vi "{{Name}}.vi"(6 "Error":errorcluster, 7 "Message":refnum<class "Message.lvclass">, 11 "ConcreteMessage":refnum<class "ConcreteMessage.lvclass">) -> (3 "ConcreteMessage":refnum<class "ConcreteMessage.lvclass">, 4 "Error":errorcluster, 5 "Message":refnum<class "Message.lvclass">)   [LabVIEW 2020, in "_Template.lvlib" / "MessageTemplate.lvlib" / "{{Name}}.lvlib" / "Message.lvclass"]
uses:
  Message.lvclass
  ConcreteMessage/ConcreteMessage.lvclass
panel:
  # "This front panel should not be manipulated."
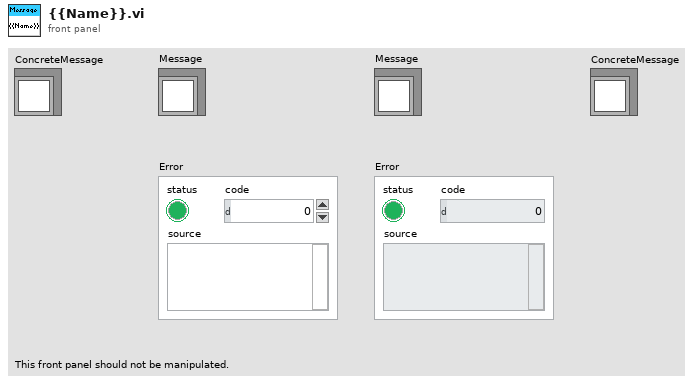
[diagram p1: front panel]
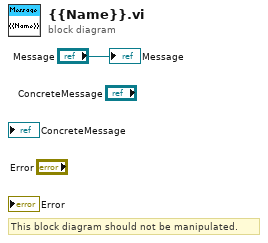
[diagram p0: block diagram]
diagram:
  # "This block diagram should not be manipulated."
  "Message" <- "Message"
